vi "经纬转换1.vi"(10 "字符串 3":string, 11 "字符串 4":string) -> (2 "字符串":string, 3 "字符串 2":string)   [LabVIEW 2015]
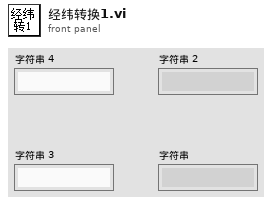
[diagram p1: front panel]
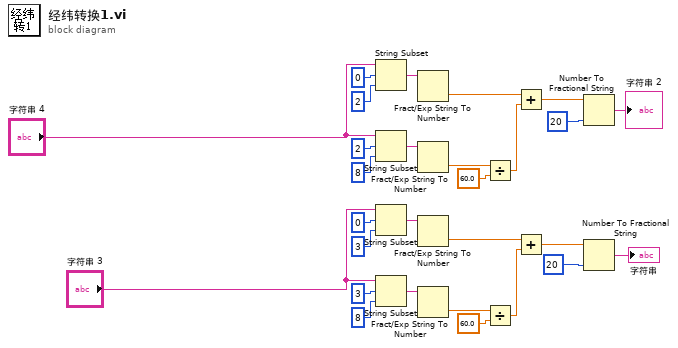
[diagram p0: block diagram]
diagram:
  n1 = String Subset(string="字符串 4", offset (0)=0 ("偏移量(0)"), length (rest)=2 ("长度（剩余）")) -> (substring=w13:string)
  n2 = String Subset(string="字符串 4", offset (0)=2 ("偏移量(0)"), length (rest)=8 ("长度（剩余）")) -> (substring=w18:string)
  n3 = String Subset(string="字符串 3", offset (0)=0 ("偏移量(0)"), length (rest)=3 ("长度（剩余）")) -> (substring=w2:string)
  n4 = String Subset(string="字符串 3", offset (0)=3 ("偏移量(0)"), length (rest)=8 ("长度（剩余）")) -> (substring=w7:string)
  n5 = Fract/Exp String To Number(string=w13) -> (number=w12:dbl)  [unwired: 3 in, 1 out]
  n6 = Fract/Exp String To Number(string=w18) -> (number=w17:dbl)  [unwired: 3 in, 1 out]
  n7 = Fract/Exp String To Number(string=w2) -> (number=w1:dbl)  [unwired: 3 in, 1 out]
  n8 = Fract/Exp String To Number(string=w7) -> (number=w6:dbl)  [unwired: 3 in, 1 out]
  n9 = Divide(x=w17, y=60.0) -> (x/y=w15:dbl)
  n10 = Divide(x=w6, y=60.0) -> (x/y=w4:dbl)
  n11 = Add(x=w12, y=w15) -> (x+y=w14:dbl)
  n12 = Add(x=w1, y=w4) -> (x+y=w3:dbl)
  n13 = Number To Fractional String(number=w14, precision (6)=i16 20 ("精度(6)")) -> (F-format string=→"字符串 2":string)  [unwired: 2 in]
  n14 = Number To Fractional String(number=w3, precision (6)=i16 20 ("精度(6)")) -> (F-format string=→"字符串":string)  [unwired: 2 in]
